vi "Intake Controller.vi"(8 "error in":errorcluster) -> ()   [LabVIEW 2017]
doc: "This VI executes continuously carrying out the current operation and responding to updates or new operations. It will often contain the timing or control code that is difficult to place directly in TeleOp. This VI generally opens all sensors and motors and isolates the rest of the robot code from knowing how the operations are carried out."
uses:
  <vilib>/Rock Robotics/WPI/Framework/Completion Status.ctl
  Intake Setpoints.ctl
  Intake Operations.ctl
  <vilib>/Rock Robotics/SystemInterfaces/DIO/FPGA_DIOPWMChannel.ctl
  <vilib>/Rock Robotics/SystemInterfaces/DIO/FPGA_DIOChannel.ctl
  <extravilib>/ChannelInstances/Lossy Stream-bool/Write With Abort.vi
  <extravilib>/ChannelInstances/Lossy Stream-bool/Read With Abort.vi
  <extravilib>/ChannelInstances/Lossy Stream-bool/Endpoint.vi
  <extravilib>/ChannelInstances/Lossy Stream-bool/EndpointRead.vi
  <vilib>/Rock Robotics/WPI/RobotDrive/WPI_RobotDriveOpen2MotorWithTalon.vi
  <vilib>/Rock Robotics/WPI/Switch/WPI_SwitchOpenLimit.vi
  <extravilib>/ChannelInstances/Lossy Stream-bool/Instantiate.vi
  <extravilib>/ChannelInstances/Lossy Stream-bool/)Channel.vi
  <resource>/ChannelSupport/_ChannelSupport/WaitIfNeeded.vi
  <vilib>/Rock Robotics/Network Tables/NT Write Boolean.vi
  <extravilib>/ChannelInstances/Lossy Stream-bool.lvlib
panel:
  out "Has Cube":bool
  in  "Interactive Values":T1
  out "Current\nCmd":string
  in  "Buttons":cluster{"Execute Cmd":bool, "Abort Cmd":bool}
  out "Command Timing":cluster{"Start Time (ms)":u32, "Iterations":i32}
  out "Status":T3
  # "Tip: It may be helpful to observe inputs and sensor values.\nYou may also want to display tuning or debugging controls."
  # "Interactive Command: You may fill in the settings for a command\nand schedule it with the Execute button. You can observe and abort\nany command while fine tuning the code for the controller."
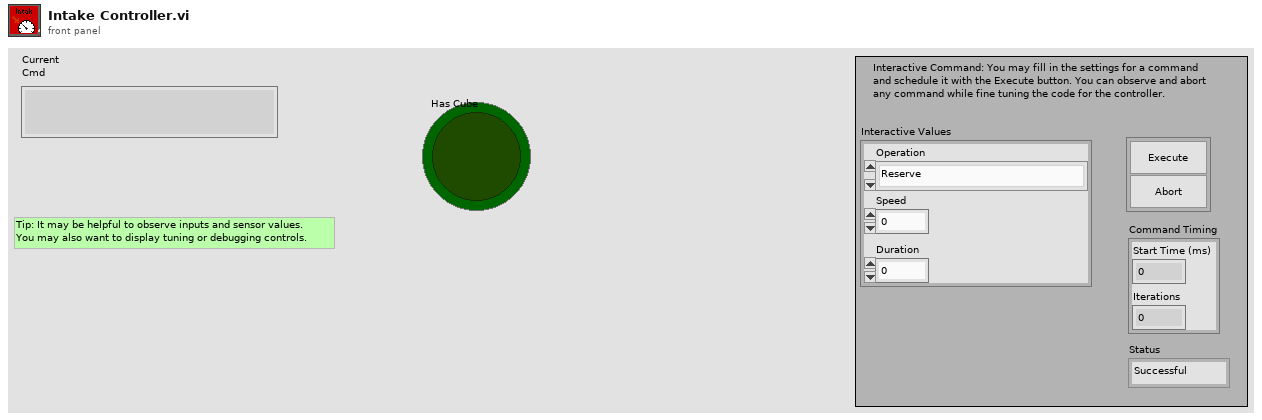
[diagram p1: front panel]
types:
  T1 = typedef "Intake Setpoints.ctl" = cluster{"Operation":T2, "Speed":dbl, "Duration":dbl}
  T2 = typedef "Intake Operations.ctl" = enum16{"Reserve", "Read Current", "Immediate", "Intake for Duration", "Intake Until Cube"}
  T3 = typedef "Completion Status.ctl" = enum16{"Successful", "Aborted", "Incomplete"}
  T4 = typedef "FPGA_DIOChannel.ctl" = enum8{"DIO 0", "DIO 1", "DIO 2", "DIO 3", "DIO 4", "DIO 5", "DIO 6", "DIO 7", "DIO 8", "DIO 9", "DIO MXP 0", "DIO MXP 1", "DIO MXP 2", "DIO MXP 3", "DIO MXP 4", "DIO MXP 5", "DIO MXP 6", "DIO MXP 7", "DIO MXP 8", "DIO MXP 9", "DIO MXP 10", "DIO MXP 11", "DIO MXP 12", "DIO MXP 13", "DIO MXP 14", "DIO MXP 15", "SPI Port CS1", "SPI Port CS2", "SPI Port CS3", "SPI Port MISO", "SPI Port MOSI", "Invalid"}
  T5 = typedef "FPGA_DIOPWMChannel.ctl" = enum8{"PWM 0", "PWM 1", "PWM 2", "PWM 3", "PWM 4", "PWM 5", "PWM 6", "PWM 7", "PWM 8", "PWM 9", "PWM MXP 0", "PWM MXP 1", "PWM MXP 2", "PWM MXP 3", "PWM MXP 4", "PWM MXP 5", "PWM MXP 6", "PWM MXP 7", "PWM MXP 8", "PWM MXP 9", "Invalid"}
  T6 = typedef "WPI_RobotDriveDevRef.ctl" = cluster{"DevStatus":errorcluster, "Motors[]":T7[], "Square Inputs":bool, "Max Output":dbl}
  T7 = typedef "WPI_MotorControlDeviceRef.ctl" = cluster{"DeviceStatus":errorcluster, "Type":T8, "PWM":cluster{"PWM Channel":T5, "DeadBand":T9}, "CAN":cluster{"Device Number":u8, "SetOutput VI Ref":variant, "GetOutput VI Ref":variant, "Enable VI Ref":variant, "Disable VI Ref":variant, "Data":variant}, "Invert":bool, "DIO PWM":cluster{"PWM \"Enable\" Channel":T5, "DIOChannel":T4, "PWM Rate":dbl}}
  T8 = typedef "WPI_MotorControlType.ctl" = enum16{"PWM", "CAN", "DIO PWM"}
  T9 = typedef "WPI_PWMDeadband.ctl" = cluster{"Name":string, "maxPositivePwm":i32, "minPositivePwm":i32, "centerPwm":i32, "maxNegativePwm":i32, "minNegativePwm":i32, "angularRange":u16}
  T10 = typedef "WPI_SwitchDevRef.ctl" = cluster{"DevStatus":errorcluster, "DIO Channel":T4, "CntIndex":T11, "Normally Closed":bool}
  T11 = typedef "FPGA_CounterCtrSystemIndex.ctl" = enum8{"Ctr 0", "Ctr 1", "Ctr 2", "Ctr 3", "Ctr 4", "Ctr 5", "Ctr 6", "Ctr 7", "Invalid"}
  T12 = typedef "Command Status Info.ctl" = cluster{"Name":string, "Status":T3, "notifier out":T13}
  T13 = typedef "Completion Notifier.ctl" = refnum<notifier>
  T14 = cluster{"Current Command":T1, "Command Timing":cluster{"Start Time (ms)":u32, "Iterations":i32}, "Command Arguments":cluster{"Command Info":T12, "Description":string, "Default Command":T1, "queue out":refnum<queue>, "Subsystem Name":string}}
  T15 = typedef "Lossy Stream-bool.lvlib/)Channel.ctl" = refnum<queue>
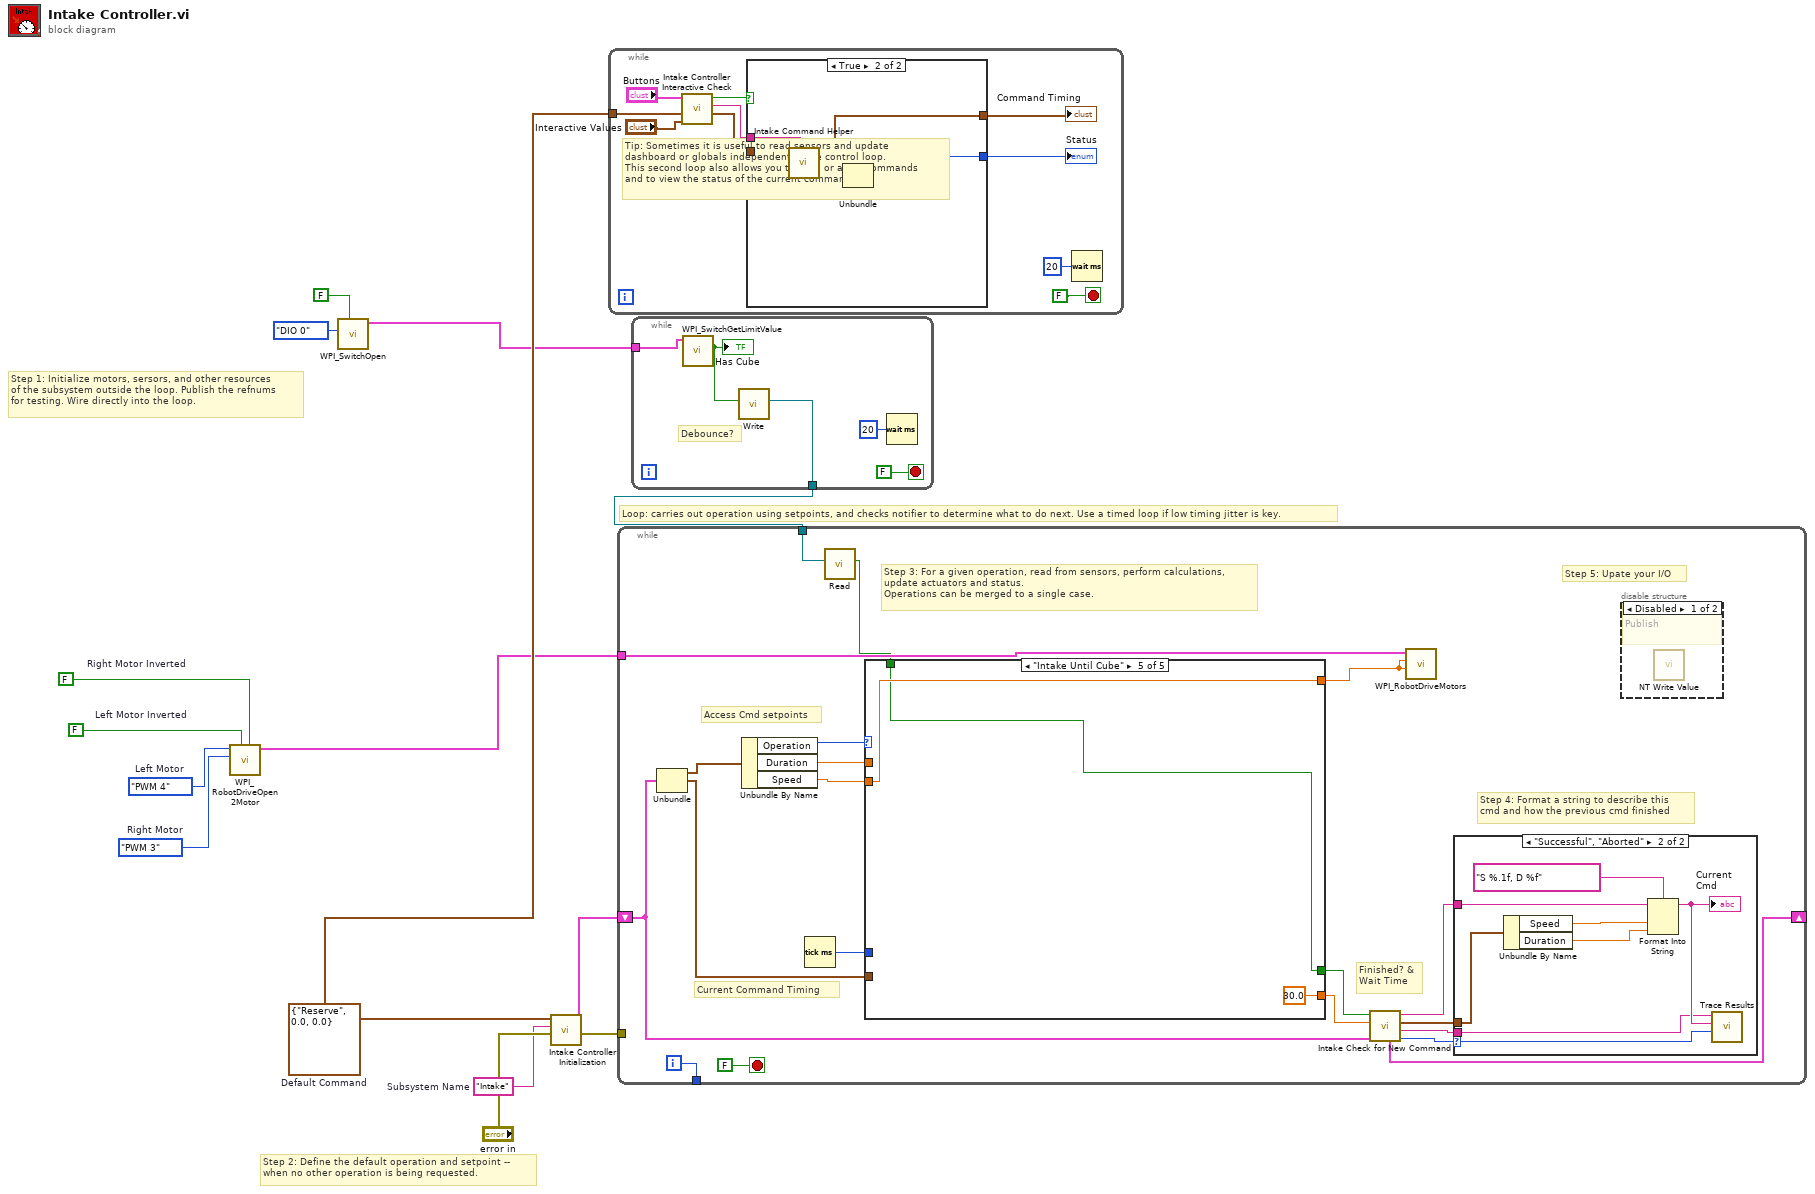
[diagram p0: block diagram]
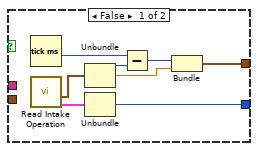
[diagram p2: hidden frame]
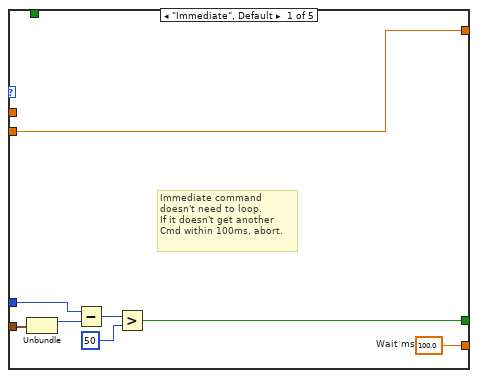
[diagram p5: hidden frame]
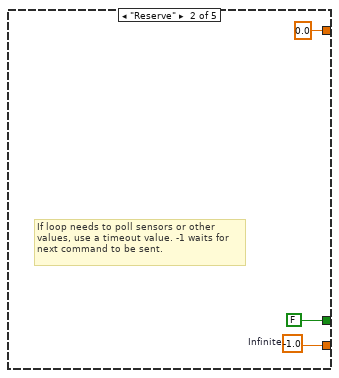
[diagram p6: hidden frame]
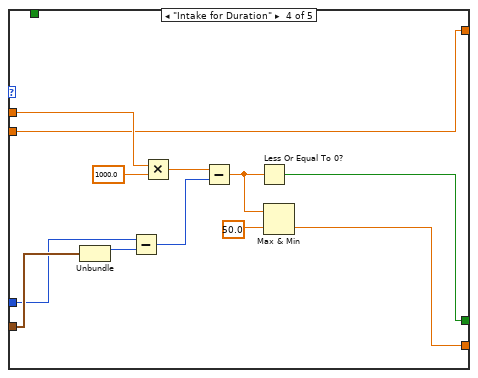
[diagram p8: hidden frame]
diagram:
  w6 = FALSE  # Right Motor Inverted
  w7 = FALSE  # Left Motor Inverted
  w8 = FPGA_DIOPWMChannel."PWM 3"  # Right Motor
  w9 = FPGA_DIOPWMChannel."PWM 4"  # Left Motor
  w10 = T1 {"Operation"=enum."Reserve", "Speed"=0.0, "Duration"=0.0}  # Default Command
  w11 = "Intake"  # Subsystem Name
  # "Tip: Sometimes it is useful to read sensors and update\ndashboard or globals independent of the control loop.\nThis second loop also allows you to send or abort commands\nand to view the status of the current command."
  # "Step 2: Define the default operation and setpoint --\nwhen no other operation is being requested."
  # "Step 1: Initialize motors, sersors, and other resources\nof the subsystem outside the loop. Publish the refnums\nfor testing. Wire directly into the loop."
  # "Loop: carries out operation using setpoints, and checks notifier to determine what to do next. Use a timed loop if low timing jitter is key."
  n1 = call-poly <vilib>:"WPI_RobotDriveOpen2Motor.vi"("Right Motor Inverted"=w6, "Left Motor Inverted"=w7, "Right Motor"=w8, "Left Motor"=w9) -> ("RobotDriveDevRef"=w5:T6)  [unwired: 6 in, 1 out]
  n2 = call-poly <vilib>:"WPI_SwitchOpen.vi"("Normally Closed"=FALSE, "DIO Channel"=FPGA_DIOChannel."DIO 0") -> ("SwitchDevRef"=w3:T10)  [unwired: 8 in, 1 out]
  n3 = call "Intake Controller Initialization.vi"("Subsystem Name"=w11, "Default Command"=w10) -> ("Current Command"=w12:T14)  [unwired: 9 in]
  n4 = while {
    tunnel: w10 -> [w20]
    stop <- FALSE stop-if-true
    n5 = call "Intake Controller Interactive Check.vi"("Interactive Command in"="Interactive Values", "Default Command"=w20, "Buttons"="Buttons") -> ("Interactive Command out"=w17:T1, "Trace String"=w18:string, "Schedule"=w19:bool)  [unwired: 6 in]
    n6 = case shown="True" w19 {
      tunnel: [w31 w36] -> w16
      tunnel: w17 -> [_ w34]
      tunnel: [w27 w32] -> w15
      tunnel: w18 -> [_ w35]
      frame False {
        n7 = Tick Count (ms)() -> (millisecond timer value=w26:u32)
        n8 = call "Read Intake Operation.vi"() -> ("Command Info"=w24:T12, "SubSystem Data"=w25:T1)  [unwired: 9 in, 1 out]
        n9 = Unbundle(w25) -> ("Operation"=w30:T2, "Speed"=w28:dbl)  [unwired: 1 out]
        n10 = Unbundle(w24) -> ("Status"=w31:T3)  [unwired: 2 out]
        n11 = Subtract(x=w26, y=w30) -> (x-y=w29:u32)
        n12 = Bundle(w29, "Speed"=w28) -> (w27:cluster{u32, "Speed":dbl})  [unwired: 1 in]
      }
      frame True {
        n13 = call "Intake Command Helper.vi"("Description"=w35, "SubSystem Data"=w34) -> ("Command Info Out"=w33:T12, "Command Timing"=w32:cluster{"Start Time (ms)":u32, "Iterations":i32})  [unwired: 7 in, 1 out]
        n14 = Unbundle(w33) -> ("Status"=w36:T3)  [unwired: 2 out]
      }
    }
    "Status" <- w16
    "Command Timing" <- w15
    n15 = Wait (ms)(milliseconds to wait=u32 20) -> ()  [unwired: 1 out]
  }
  n16 = while {
    tunnel: w3 -> [w40]
    tunnel: [w38] -> w1
    stop <- FALSE stop-if-true
    # "Debounce?"
    n17 = call <vilib>:"WPI_SwitchGetLimitValue.vi"("SwitchDevRef"=w40) -> ("Switch Pressed"=w39:bool)  [unwired: 8 in, 2 out]
    "Has Cube" <- w39
    n18 = call <extravilib>:"Write.vi"("element"=w39) -> ("channel"=w38:T15)  [unwired: 8 in, 2 out]
    n19 = Wait (ms)(milliseconds to wait=u32 20) -> ()  [unwired: 1 out]
  }
  n20 = while {
    shift-right: [w53] -> _
    shift-left: w12 -> [w46]
    tunnel: [w60] -> _
    tunnel: "error in" -> [_]
    tunnel: w5 -> [w45]
    tunnel: w1 -> [w43]
    i -> [w60]
    stop <- FALSE stop-if-true
    # "Step 5: Upate your I/O"
    # "Step 4: Format a string to describe this\ncmd and how the previous cmd finished"
    # "Current Command Timing"
    # "Access Cmd setpoints"
    # "Finished? &\nWait Time"
    # "Step 3: For a given operation, read from sensors, perform calculations,\nupdate actuators and status.\nOperations can be merged to a single case."
    n21 = Unbundle(w46) -> ("Current Command"=w59:T1, "Command Timing"=w55:cluster{"Start Time (ms)":u32, "Iterations":i32})  [unwired: 1 out]
    n22 = Unbundle By Name(w59) -> ("Operation"=w58:T2, "Duration"=w57:dbl, "Speed"=w54:dbl)
    n23 = Tick Count (ms)() -> (millisecond timer value=w56:u32)
    n24 = call <extravilib>:"Read.vi"("channel"=w43) -> ("element"=w42:bool)  [unwired: 5 in, 5 out]
    n25 = case shown="\"Intake Until Cube\"" w58 {
      tunnel: [w77 w80 _ w83 30.0 ("Infinite")] -> w51
      tunnel: [w71 FALSE ("ignore previous (F)") _ w84 w93] -> w52
      tunnel: w55 -> [w73 _ _ w82 _]
      tunnel: w57 -> [_ _ _ w86 _]
      tunnel: w56 -> [w72 _ _ w81 _]
      tunnel: w54 -> [w70 _ _ w85 w95]
      tunnel: [w70 0.0 ("Speed") _ w85 w95] -> w44
      tunnel: w42 -> [_ _ _ _ w93]
      frame "Immediate", Default {
        w77 = 100.0  # Wait ms
        # "Immediate command\ndoesn't need to loop.\nIf it doesn't get another\nCmd within 100ms, abort."
        n26 = Unbundle(w73) -> ("Start Time (ms)"=w76:u32)  [unwired: 1 out]
        n27 = Subtract(x=w72, y=w76) -> (x-y=w75:u32)
        n28 = Greater?(x=w75, y=u8 50 ("Left Motor")) -> (0:w71:bool)
      }
      frame "Reserve" {
        w80 = -1.0  # Infinite
        # "If loop needs to poll sensors or other\nvalues, use a timeout value. -1 waits for\nnext command to be sent."
      }
      frame "Read Current" {
      }
      frame "Intake for Duration" {
        n29 = Unbundle(w82) -> ("Start Time (ms)"=w89:u32)  [unwired: 1 out]
        n30 = Subtract(x=w81, y=w89) -> (x-y=w92:u32)
        n31 = Multiply(x=w86, y=1000.0) -> (x*y=w91:dbl)
        n32 = Subtract(x=w91, y=w92) -> (x-y=w88:dbl)
        n33 = Less Or Equal To 0?(x=w88) -> (x <= 0?=w84:bool)
        n34 = Max & Min(x=w88, y=50.0) -> (min(x,y)=w83:dbl)  [unwired: 1 out]
      }
      frame "Intake Until Cube" {
      }
    }
    n35 = call "Intake Check for New Command.vi"("Current Command"=w46, "Wait time (ms)"=w51, "Finished?"=w52) -> ("Completion"=w47:T3, "Subsystem Name"=w48:string, "Current Command"=w49:T1, "Initial Trace String"=w50:string, "NextCommand"=w53:T14)  [unwired: 4 in]
    n36 = call <vilib>:"WPI_RobotDriveMotors.vi"("RightSpeed"=w44, "LeftSpeed"=w44, "RobotDriveDevRef"=w45) -> ()  [unwired: 1 in, 8 out]
    n37 = case shown="\"Successful\", \"Aborted\"" w47 {
      selector: w47 -> [_ w69]
      tunnel: w50 -> [_ w65]
      tunnel: w49 -> [_ w66]
      tunnel: w48 -> [_ w62]
      frame "Incomplete", Default {
        # "Continuing current command"
      }
      frame "Successful", "Aborted" {
        # "Report and setup for next command"
        n38 = Unbundle By Name(w66) -> ("Speed"=w68:dbl, "Duration"=w63:dbl)
        n39 = Format Into String(format string="S %.1f, D %f", initial string=w65, w68, w63) -> (resulting string=w64:string)  [unwired: 1 in, 1 out]
        "Current\nCmd" <- w64
        n40 = call <vilib>:"Trace Results.vi"("Status of previous command"=w69, "Description"=w64, "Subsystem"=w62) -> ()  [unwired: 9 in]
      }
    }
    n41 = disable-structure shown="Disabled" {
      frame Disabled {
        # "Publish"
        n42 = call-poly <vilib>:"NT Write Value.vi"() -> ()  [unwired: 11 in, 1 out]
      }
      frame Enabled {
      }
    }
  }
